vi "Write Test Report.vi"(10 "Test Report":refnum<class "Test Report.lvclass">, 11 "Test Runner in":refnum<class "Test Runner.lvclass">) -> (3 "Test Runner out":refnum<class "Test Runner.lvclass">)   [LabVIEW 2013, in "Caraya.lvlib" / "Test Runner.lvclass"]
uses:
  Test Runner.lvclass
  Test Report/Test Report.lvclass
  Test Runner.lvclass/Test Runner.ctl
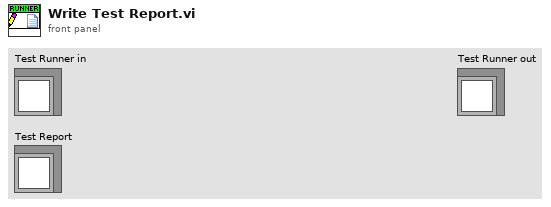
[diagram p1: front panel]
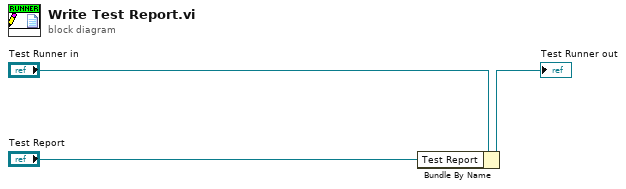
[diagram p0: block diagram]
diagram:
  n1 = Bundle By Name(cluster="Test Runner in", "Test Report"="Test Report") -> (→"Test Runner out":refnum<class "Test Runner.lvclass">)
